vi "DriverStationGetData.vi"   [LabVIEW 2020]
doc: "This VI recieves data from the FRC 4265 Dashboard continuously, in all robot modes. These may include safety overrides, calibration commands, and configuration parameters. However this VI should never include standard driver or manipulator commands."
uses:
  <vilib>/Rock Robotics/Network Tables/NT Read String.vi
  dsdata.vi
  <vilib>/Rock Robotics/Network Tables/NT Read Number.vi
  refnums.vi
  GRNF_Joystick.vi
types:
  T1 = typedef "WPI_JoystickDevRef.ctl" = cluster{"Device":T2}
  T2 = typedef "WPI_JoystickDeviceEnum.ctl" = enum16{"USB 0", "USB 1", "USB 2", "USB 3", "USB 4", "USB 5"}
  T3 = enum16{"Center", "North", "NorthWest", "West", "SouthWest", "South", "SouthEast", "East", "NorthEast"}
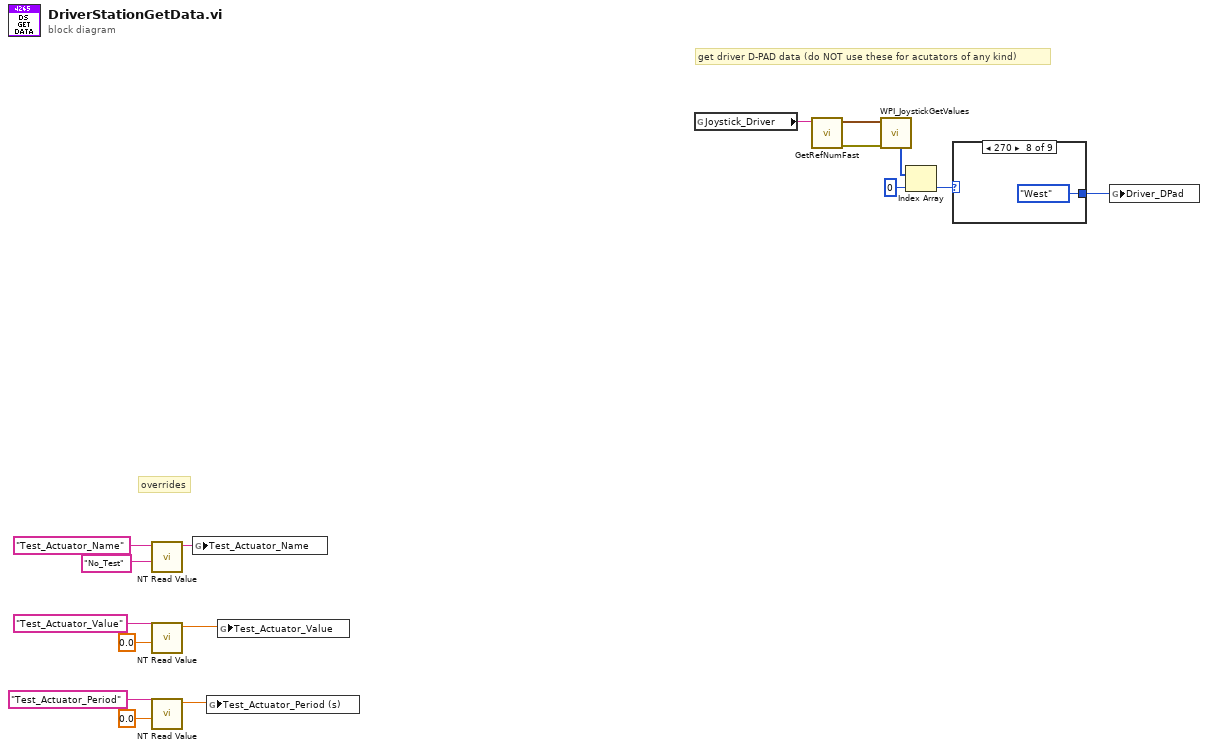
[diagram p0: block diagram]
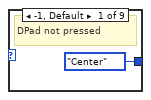
[diagram p2: hidden frame]
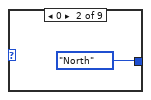
[diagram p3: hidden frame]
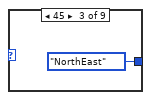
[diagram p4: hidden frame]
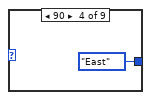
[diagram p5: hidden frame]
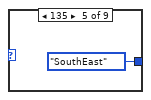
[diagram p6: hidden frame]
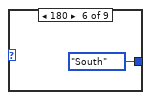
[diagram p7: hidden frame]
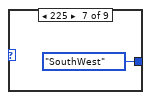
[diagram p8: hidden frame]
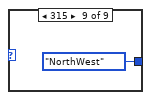
[diagram p9: hidden frame]
diagram:
  # "get driver D-PAD data (do NOT use these for acutators of any kind)"
  # "overrides"
  n1 = call-poly <vilib>:"NT Read Value.vi"("Default Value"="No_Test", "Name"="Test_Actuator_Name" ("refnum name")) -> ("String"=w15:string)  [unwired: 8 in, 1 out]
  n2 = call-poly <vilib>:"NT Read Value.vi"("Default Value"=0.0, "Name"="Test_Actuator_Value" ("refnum name")) -> ("Numeric"=w11:dbl)  [unwired: 8 in, 1 out]
  n3 = call-poly <vilib>:"NT Read Value.vi"("Default Value"=0.0, "Name"="Test_Actuator_Period" ("refnum name")) -> ("Numeric"=w9:dbl)  [unwired: 8 in, 1 out]
  n4 = global write "dsdata.vi" "Test_Actuator_Name"(w15) -> ()
  n5 = global write "dsdata.vi" "Test_Actuator_Period (s)"(w9) -> ()
  n6 = global write "dsdata.vi" "Test_Actuator_Value"(w11) -> ()
  n7 = global read "refnums.vi" "Joystick_Driver"() -> (w5:string)
  n8 = call-poly "GetRefNumFast.vi"("RefNum Name"=w5) -> ("Error"=w6:errorcluster, "Device Reference"=w7:T1)  [unwired: 5 in]
  n9 = call <vilib>:"WPI_JoystickGetValues.vi"("error in (no error)"=w6, "JoystickDevRef"=w7) -> ("POVs"=w2:i16[])  [unwired: 5 in, 4 out]
  n10 = Index Array(array=w2, index=0) -> (element=w3:i16)
  n11 = case shown="270" w3 {
    tunnel: [T3."Center" T3."North" T3."NorthEast" T3."East" T3."SouthEast" T3."South" T3."SouthWest" T3."West" T3."NorthWest"] -> w1
    frame -1, Default {
      # "DPad not pressed"
    }
    frame 0 {
    }
    frame 45 {
    }
    frame 90 {
    }
    frame 135 {
    }
    frame 180 {
    }
    frame 225 {
    }
    frame 270 {
    }
    frame 315 {
    }
  }
  n12 = global write "dsdata.vi" "Driver_DPad"(w1) -> ()
